vi "LVRT Serial Write.vi"(8 "error in (no error)":errorcluster, 10 "String":string="*IDN?\n", 11 "FPGA Main Ref":refnum<k20>) -> (0 "error out":errorcluster, 3 "FPGA Main Ref Out":refnum<k20>)   [LabVIEW 2014]
uses:
  <vilib>/Utility/error.llb/Error Cluster From Error Code.vi
  <vilib>/rvi/errors/niLvFpgaAdjustHostInterfaceError.vi
  <vilib>/rvi/interface/nirviReadWriteControl/nirviReadWriteControl.xnode
  FPGA Bitfiles/myRIOMidiIn_FPGATarget_FPGAMain_ATizAUb0m2E.lvbitx
  FPGA Main.vi
  NiFpgaLv.dll
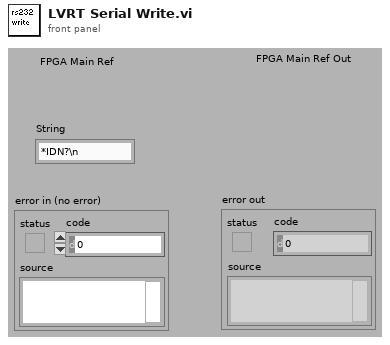
[diagram p1: front panel]
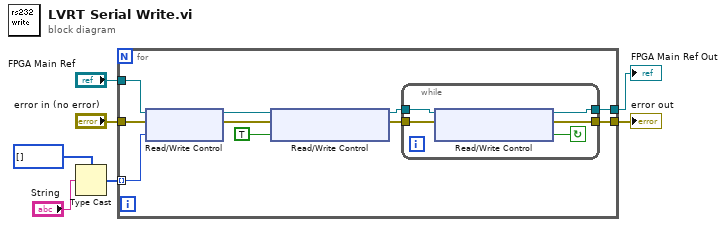
[diagram p0: block diagram]
diagram:
  n1 = Type Cast(type=u8[] [], x="String") -> (*(type *) &x=w4:u8[])
  n2 = for {
    tunnel: "FPGA Main Ref" -> [w14]
    tunnel: [w9] -> w2
    tunnel: "error in (no error)" -> [w13]
    tunnel: [w8] -> w1
    tunnel: w4 -> [w15] mode=indexing
    n3 = xnode "Read/Write Control"("FPGA VI Reference In"=w14, "error in"=w13, "Write: Char"=w15) -> ("FPGA VI Reference Out"=w17:refnum<k20>, "error out"=w16:errorcluster)
    n4 = xnode "Read/Write Control"("FPGA VI Reference In"=w17, "error in"=w16, "Write: Data Written"=TRUE ("Data Read")) -> ("FPGA VI Reference Out"=w11:refnum<k20>, "error out"=w10:errorcluster)
    n5 = while {
      tunnel: w11 -> [w22]
      tunnel: w10 -> [w21]
      tunnel: [w20] -> w9
      tunnel: [w19] -> w8
      stop <- w18 continue-if-true
      n6 = xnode "Read/Write Control"("FPGA VI Reference In"=w22, "error in"=w21) -> ("FPGA VI Reference Out"=w20:refnum<k20>, "error out"=w19:errorcluster, "Write: Data Written"=w18:bool)
    }
  }
  "error out" <- w1
  "FPGA Main Ref Out" <- w2
